vi "Pause.vi"(8 "error in (no error)":errorcluster, 11 "SR430Class in":refnum<class "SR430Class.lvclass">) -> (0 "error out":errorcluster, 3 "SR430Class out":refnum<class "SR430Class.lvclass">)   [LabVIEW 2015, in "SR430Class.lvclass"]
uses:
  class/SR430Class.lvclass
  class/SR430Class.lvclass/SR430Class.ctl
  support/SR430 Driver/SR430Driver.lvlib
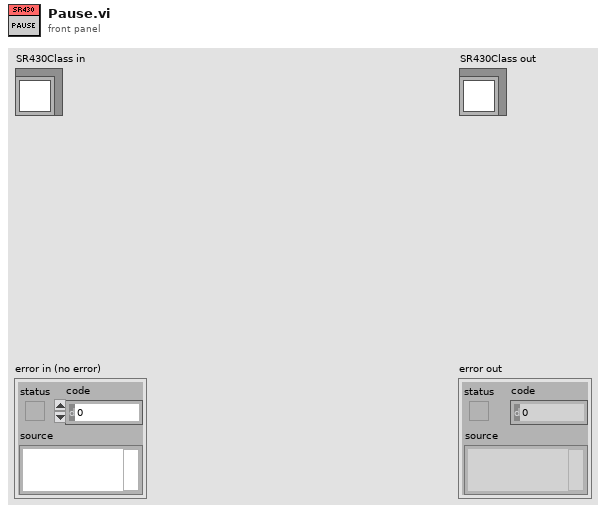
[diagram p1: front panel]
types:
  T1 = typedef "SR430Driver.lvlib/SR430_VISA Control.ctl" = cluster{"VISA resource name":refnum<visa-resource-name>}
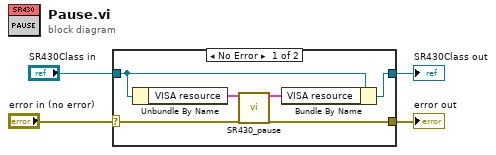
[diagram p0: block diagram]
diagram:
  n1 = case shown="No Error" "error in (no error)" {
    selector: "error in (no error)" -> [w6 w12]
    tunnel: [w5 w12] -> w3
    tunnel: [w7 w11] -> w1
    tunnel: "SR430Class in" -> [w10 w11]
    frame No Error {
      n2 = Unbundle By Name(w10) -> ("VISA resource"=w9:T1)
      n3 = call "SR430_pause.vi"("address"=w9, "error in (no error)"=w6) -> ("address out"=w8:T1, "error out"=w5:errorcluster)  [unwired: 16 in]
      n4 = Bundle By Name(cluster=w10, "VISA resource"=w8) -> (w7:refnum<class "SR430Class.lvclass">)
    }
    frame Error {
    }
  }
  "error out" <- w3
  "SR430Class out" <- w1
